vi "_XNET Convert List From Array To Comma.vi"(7 "error in (no error)":errorcluster, 10 "list in":string[](array[string])) -> (0 "error out":errorcluster, 1 "commaSeparatedList out":string, 2 "cluster out":string, 3 "database out":string)   [LabVIEW 2018]
doc: "Internal subVI of NI-XNET.\n\nThe NI-XNET driver uses ASCIIZ strings in which multiple items are separated by comma. This subVI takes an array of database I/O names (each using the database selection suffix), and forms a list of comma-separated names for the NI-XNET driver."
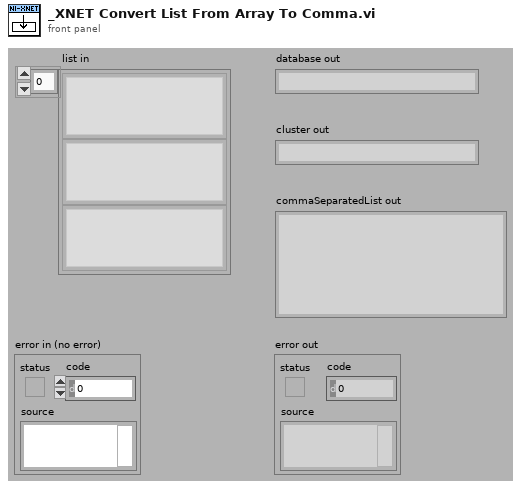
[diagram p1: front panel]
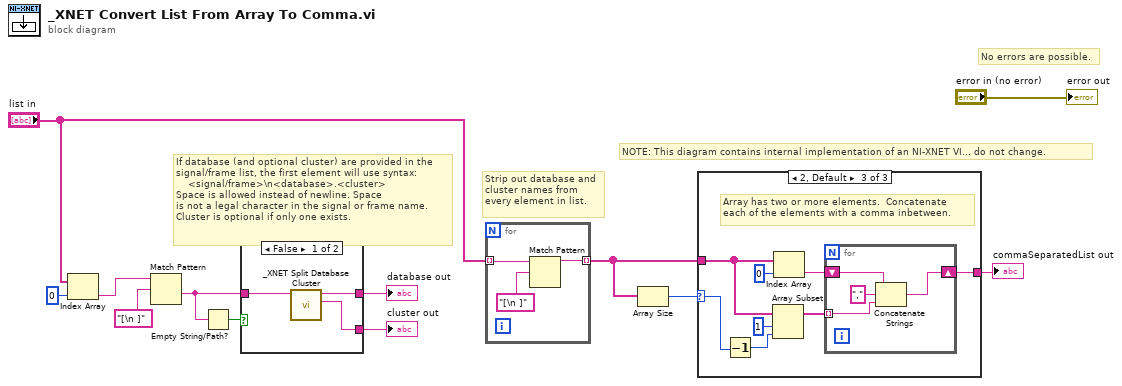
[diagram p0: block diagram]
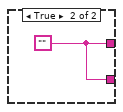
[diagram p2: hidden frame]
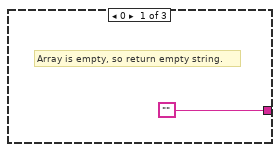
[diagram p3: hidden frame]
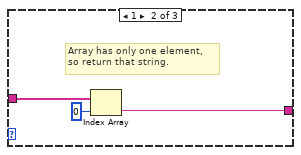
[diagram p4: hidden frame]
diagram:
  # "Strip out database and\ncluster names from \nevery element in list."
  # "If database (and optional cluster) are provided in the\nsignal/frame list, the first element will use syntax:\n    <signal/frame>\\n<database>.<cluster>\nSpace is allowed instead of newline. Space\nis not a legal character in the signal or frame name.\nCluster is optional if only one exists."
  # "No errors are possible."
  # "NOTE: This diagram contains internal implementation of an NI-XNET VI... do not change."
  n1 = Index Array(array="list in", index=0) -> (element=w8:string)
  n2 = Match Pattern(string=w8, regular expression="[\n ]") -> (after substring=w4:string)  [unwired: 4 out]
  n3 = Empty String/Path?(string/path=w4) -> (empty?=w6:bool)
  n4 = case shown="False" w6 {
    tunnel: w4 -> [w15 _]
    tunnel: [w14 w16] -> w5
    tunnel: [w13 w16] -> w3
    frame False {
      n5 = call "_XNET Split Database Cluster.vi"("database cluster"=w15) -> ("cluster"=w13:string, "database"=w14:string)  [unwired: 1 in, 7 out]
    }
    frame True {
      w16 = ""
    }
  }
  "database out" <- w5
  "cluster out" <- w3
  n6 = for {
    tunnel: "list in" -> [w18] mode=indexing
    tunnel: [w17] -> w1 mode=indexing
    n7 = Match Pattern(string=w18, regular expression="[\n ]") -> (before substring=w17:string)  [unwired: 4 out]
  }
  n8 = Array Size(array=w1) -> (size(s)=w12:i32)
  n9 = case shown="2, Default" w12 {
    selector: w12 -> [_ _ w26]
    tunnel: ["" w21 w30] -> w10
    tunnel: w1 -> [_ w22 w24]
    frame 0 {
      # "Array is empty, so return empty string."
    }
    frame 1 {
      # "Array has only one element, \nso return that string."
      n10 = Index Array(array=w22, index=0 ("Index")) -> (element=w21:string)
    }
    frame 2, Default {
      # "Array has two or more elements.  Concatenate\neach of the elements with a comma inbetween."
      n11 = Decrement(x=w26) -> (x-1=w27:i32)
      n12 = Array Subset(array=w24, index=1 ("Array Index"), length=w27) -> (w29:string[])
      n13 = Index Array(array=w24, index=0 ("Index")) -> (element=w25:string)
      n14 = for {
        tunnel: w29 -> [w32] mode=indexing
        shift-right: [w33] -> w30
        shift-left: w25 -> [w34]
        n15 = Concatenate Strings(w34, "," ("Substring"), w32) -> (w33:string)
      }
    }
  }
  "commaSeparatedList out" <- w10
  "error out" <- "error in (no error)"
